vi "Память.vi"(0 "Inp":T2, 1 "Adr A":cluster{"a0":bool, "a1":bool}, 2 "Adr b":cluster{"a0":bool, "a1":bool}, 3 "c":bool, 4 "wr":bool) -> (5 "A":T1, 6 "B":T1)   [LabVIEW 2013]
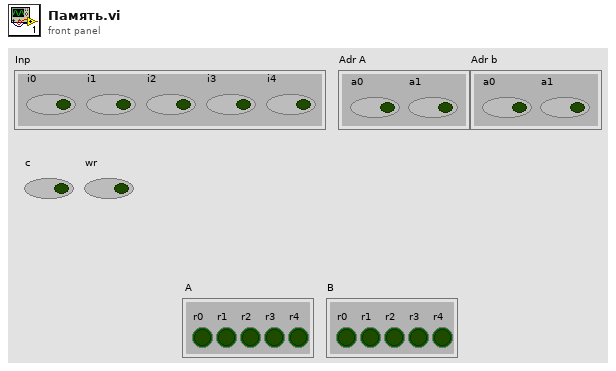
[diagram p1: front panel]
types:
  T1 = cluster{"r0":bool, "r1":bool, "r2":bool, "r3":bool, "r4":bool}
  T2 = cluster{"i0":bool, "i1":bool, "i2":bool, "i3":bool, "i4":bool}
  T3 = cluster{"q4":bool, "q3":bool, "q2":bool, "q1":bool, "q0":bool}
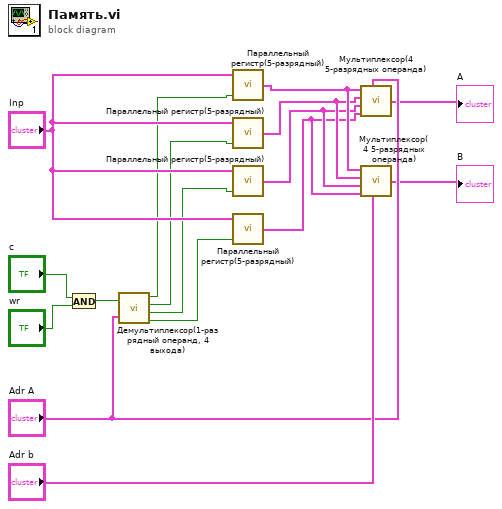
[diagram p0: block diagram]
diagram:
  n1 = And(x="c", y="wr") -> (x .and. y?=w13:bool)
  n2 = call "Демультиплексор(1-разрядный операнд, 4 выхода).vi"("a"=w13, "c"="Adr A") -> ("r0"=w12:bool, "r1"=w11:bool, "r2"=w10:bool, "r3"=w9:bool)
  n3 = call "Параллельный регистр(5-разрядный).vi"("C"=w12, "Cluster"="Inp") -> ("output cluster"=w8:T3)  [unwired: 1 in]
  n4 = call "Параллельный регистр(5-разрядный).vi"("C"=w11, "Cluster"="Inp") -> ("output cluster"=w7:T3)  [unwired: 1 in]
  n5 = call "Параллельный регистр(5-разрядный).vi"("C"=w10, "Cluster"="Inp") -> ("output cluster"=w6:T3)  [unwired: 1 in]
  n6 = call "Параллельный регистр(5-разрядный).vi"("C"=w9, "Cluster"="Inp") -> ("output cluster"=w5:T3)  [unwired: 1 in]
  n7 = call "Мультиплексор(4 5-разрядных операнда).vi"("Inp0"=w8, "Inp1"=w7, "Inp2"=w6, "Inp3"=w5, "с"="Adr A") -> ("r"=→"A":T1)
  n8 = call "Мультиплексор(4 5-разрядных операнда).vi"("Inp0"=w8, "Inp1"=w7, "Inp2"=w6, "Inp3"=w5, "с"="Adr b") -> ("r"=→"B":T1)
